vi "Working beep.vi"   [LabVIEW 2017]
uses:
  <vilib>/measure/NI_MABase.lvlib
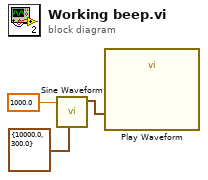
[diagram p0: block diagram]
diagram:
  n1 = call <vilib>:"Sine Waveform.vi"("sampling info"=cluster{"Fs":dbl, "#s":dbl} {"Fs"=10000.0, "#s"=300.0}, "frequency"=1000.0) -> ("signal out"=w1:waveform(dbl))  [unwired: 8 in, 1 out]
  n2 = call "Play Waveform"("Data"=w1) -> ()  [unwired: 18 in, 1 out]
